vi "Anti Intergral Windup.vi"(7 "Disable":bool, 9 "|Limit|":dbl, 10 "MV":dbl, 11 "PID gains":T1={"proportional gain (Kc)"=1.0, "integral time (Ti, min)"=0.01, "derivative time (Td, min)"=0.0} {"derivative time (Td, min)" format="%.3f"; "integral time (Ti, min)" format="%.3f"; "proportional gain (Kc)" format="%.3f"}) -> (3 "PID gains":T1={"proportional gain (Kc)"=1.0, "integral time (Ti, min)"=0.01, "derivative time (Td, min)"=0.0} {"derivative time (Td, min)" format="%.3f"; "integral time (Ti, min)" format="%.3f"; "proportional gain (Kc)" format="%.3f"})   [LabVIEW 2014]
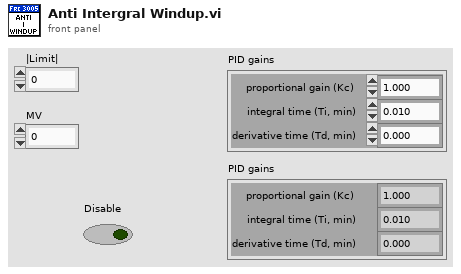
[diagram p1: front panel]
types:
  T1 = cluster{"proportional gain (Kc)":dbl, "integral time (Ti, min)":dbl, "derivative time (Td, min)":dbl}
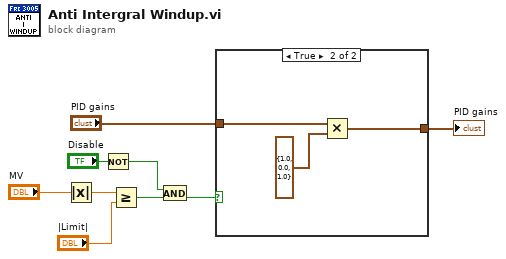
[diagram p0: block diagram]
diagram:
  n1 = Absolute Value(x="MV") -> (abs(x)=w8:dbl)
  n2 = Not(x="Disable") -> (.not. x?=w1:bool)
  n3 = Greater Or Equal?(x=w8, y="|Limit|") -> (x >= y?=w6:bool)
  n4 = And(x=w1, y=w6) -> (x .and. y?=w2:bool)
  n5 = case shown="True" w2 {
    tunnel: "PID gains" -> [w10 w13]
    tunnel: [w10 w11] -> w4
    frame False {
    }
    frame True {
      n6 = Multiply(x=w13, y=T1 {"proportional gain (Kc)"=1.0, "integral time (Ti, min)"=0.0, "derivative time (Td, min)"=1.0}) -> (x*y=w11:T1)
    }
  }
  "PID gains" <- w4
